vi "Read configuration.vi"(8 "error in":errorcluster, 11 "alarms module editor node in":refnum<class "alarms module editor node.lvclass">) -> (0 "error out":errorcluster, 2 "configuration":refnum<class "NISE_CEF_serializable configuration.lvclass">, 3 "alarms module editor node out":refnum<class "alarms module editor node.lvclass">)   [LabVIEW 2013, in "alarms module editor node.lvclass"]
uses:
  alarms module editor node.lvclass
  <vilib>/NI/Configuration Framework/serializable configuration/NISE_CEF_serializable configuration.lvclass
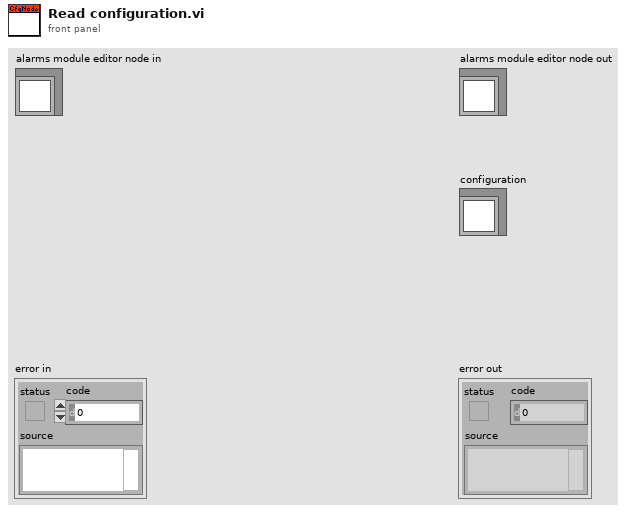
[diagram p1: front panel]
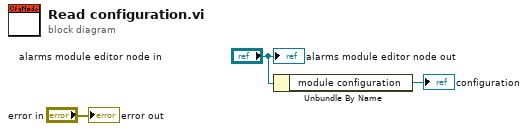
[diagram p0: block diagram]
diagram:
  n1 = Unbundle By Name("alarms module editor node in") -> ("module configuration"=→"configuration":refnum<class "alarms module configuration.lvclass">)
  "error out" <- "error in"
  "alarms module editor node out" <- "alarms module editor node in"
